vi "Write Waveform File Header.vi"(4 "Data Type":T1(ring)=enum."float64", 5 "Block Interval":dbl, 6 "File Type ID":string="WFM", 7 "Start Time":dbl, 8 "Error In":errorcluster, 9 "Sample Interval":dbl, 10 "No. of Channels":i32, 11 "File Refnum In":refnum<file>) -> (0 "Error Out":errorcluster, 3 "File Refnum Out":refnum<file>)   [LabVIEW 2015]
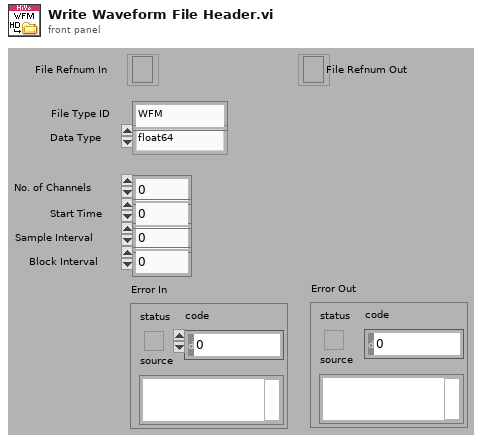
[diagram p1: front panel]
types:
  T1 = enum16{"int8", "int16", "int32", "uint8", "uint16", "uint32", "float32", "float64"}
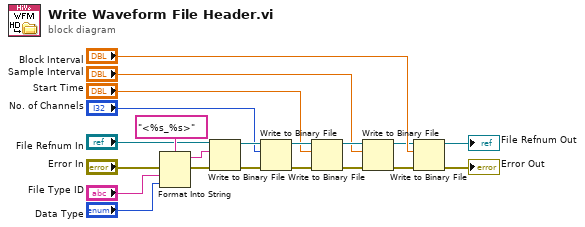
[diagram p0: block diagram]
diagram:
  n1 = Format Into String(format string="<%s_%s>", error in="Error In", "File Type ID", "Data Type") -> (resulting string=w11:string, error out=w18:errorcluster)  [unwired: 1 in]
  n2 = Write to Binary File(file (use dialog)="File Refnum In", data=w11, error in=w18) -> (refnum out=w13:refnum<file>, error out=w12:errorcluster)  [unwired: 3 in, 1 out]
  n3 = Write to Binary File(file (use dialog)=w13, data="No. of Channels", error in=w12) -> (refnum out=w14:refnum<file>, error out=w16:errorcluster)  [unwired: 3 in, 1 out]
  n4 = Write to Binary File(file (use dialog)=w14, data="Start Time", error in=w16) -> (refnum out=w15:refnum<file>, error out=w17:errorcluster)  [unwired: 3 in, 1 out]
  n5 = Write to Binary File(file (use dialog)=w15, data="Sample Interval", error in=w17) -> (refnum out=w20:refnum<file>, error out=w19:errorcluster)  [unwired: 3 in, 1 out]
  n6 = Write to Binary File(file (use dialog)=w20, data="Block Interval", error in=w19) -> (refnum out=→"File Refnum Out":refnum<file>, error out=→"Error Out":errorcluster)  [unwired: 3 in, 1 out]
